vi "ProgressPopupWithStatus_Close.vi"(8 "error in":errorcluster) -> (0 "error out":errorcluster)   [LabVIEW 2020, in "hse-ui.lvlib"]
doc: "Closes the modal progress window.\n\n\n\n____\nHAMPEL SOFTWARE ENGINEERING v3.8.0 (2023-12-18 14:41)"
uses:
  hse-ui.lvlib
  ProgressPopupWithStatus.vi
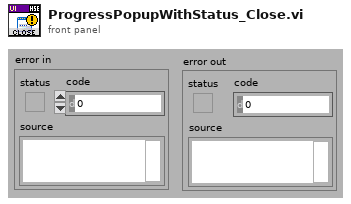
[diagram p1: front panel]
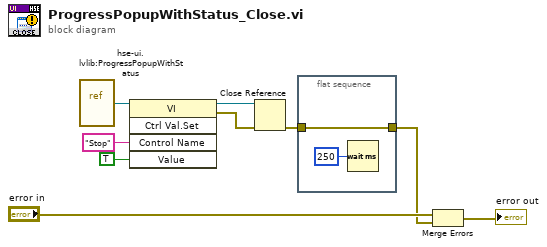
[diagram p0: block diagram]
diagram:
  n1 = vi-ref "hse-ui.lvlib:ProgressPopupWithStatus.vi"() -> (w1:refnum<vi>)
  n2 = invoke class="VI" method="Ctrl Val.Set"(reference=w1, "Control Name"="Stop", "Value"=TRUE) -> (reference out=w8:refnum<vi>, error out=w9:errorcluster)  [unwired: 2 in, 3 out]
  n3 = Close Reference(reference=w8, error in (no error)=w9) -> (error out=w5:errorcluster)
  n4 = flat-sequence {
    tunnel: w5 -> [w11]
    tunnel: [w11] -> w2
    frame #0 {
      n5 = Wait (ms)(milliseconds to wait=u32 250) -> ()  [unwired: 1 out]
    }
  }
  n6 = Merge Errors("error in", w2) -> (→"error out":errorcluster)
